vi "mod_Generate Histogram.vi"(0 "samples in":dbl[](array[numeric]) format="%.2f", 5 "max bin":dbl format="%.2f", 7 "min bin":dbl format="%.2f", 9 "bin size":dbl format="%.2f", 11 "error in (no error)":errorcluster, 13 "reset? (T)":bool=TRUE) -> (4 "histogram out":i32[](array[numeric]), 15 "error out":errorcluster)   [LabVIEW 2020, in "niAMT.lvlib"]
doc: "(c) Copyright 2006, National Instruments, Inc. This VI may not be duplicated, sold, or distributed without written consent from National Instruments."
uses:
  <vilib>/addons/Modulation/niAMT.lvlib
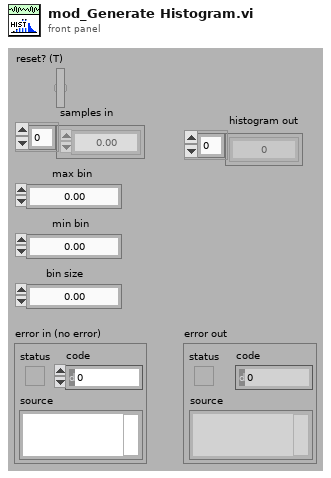
[diagram p1: front panel]
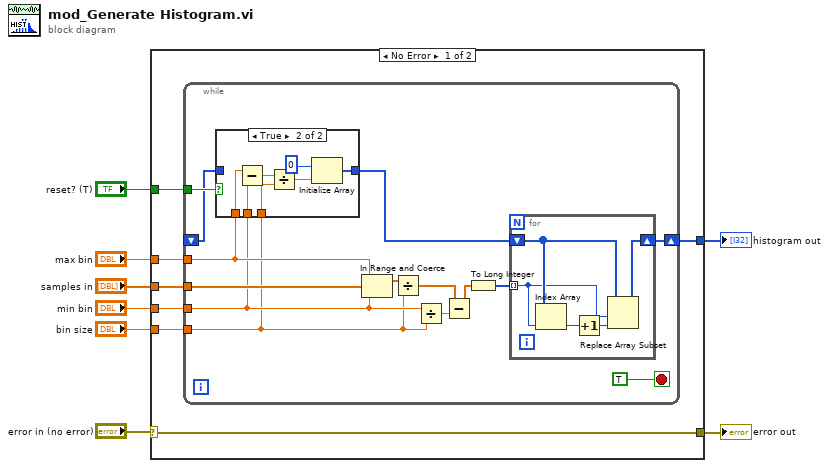
[diagram p0: block diagram]
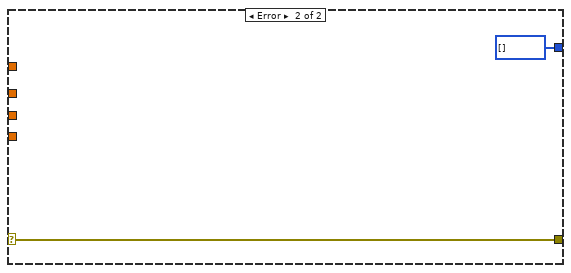
[diagram p3: hidden frame]
diagram:
  n1 = case shown="No Error" "error in (no error)" {
    selector: "error in (no error)" -> [w9 w44]
    tunnel: "samples in" -> [w15 _]
    tunnel: "min bin" -> [w14 _]
    tunnel: "max bin" -> [w13 _]
    tunnel: "bin size" -> [w12 _]
    tunnel: [w11 i32[] []] -> w4
    tunnel: "reset? (T)" -> [w10 _]
    tunnel: [w9 w44] -> w1
    frame No Error {
      n2 = while {
        tunnel: w15 -> [w29]
        tunnel: w14 -> [w20]
        tunnel: w13 -> [w21]
        tunnel: w12 -> [w19]
        shift-right: [w28] -> w11
        shift-left: _ -> [w17]
        tunnel: w10 -> [w22]
        stop <- TRUE stop-if-true
        n3 = case shown="True" w22 {
          tunnel: w21 -> [_ w34]
          tunnel: w20 -> [_ w33]
          tunnel: w19 -> [_ w32]
          tunnel: [w30 w31] -> w18
          tunnel: w17 -> [w30 _]
          frame False {
          }
          frame True {
            n4 = Subtract(x=w34, y=w33) -> (x-y=w36:dbl)
            n5 = Divide(x=w36, y=w32) -> (x/y=w35:dbl)
            n6 = Initialize Array(0 ("Numeric"), w35) -> (w31:i32[])
          }
        }
        n7 = In Range and Coerce(upper limit=w21, x=w29, lower limit=w20) -> (coerced(x)=w27:dbl[])  [unwired: 1 out]
        n8 = Divide(x=w27, y=w19) -> (x/y=w24:dbl[])
        n9 = Divide(x=w20, y=w19) -> (x/y=w25:dbl)
        n10 = Subtract(x=w24, y=w25) -> (x-y=w23:dbl[])
        n11 = To Long Integer(number=w23) -> (32bit integer=w26:i32[])
        n12 = for {
          tunnel: w26 -> [w38] mode=indexing
          shift-right: [w39] -> w28
          shift-left: w18 -> [w40]
          n13 = Index Array(array=w40, index=w38) -> (element=w42:i32)
          n14 = Increment(x=w42) -> (x+1=w41:i32)
          n15 = Replace Array Subset(array=w40, new element=w41, index=w38) -> (w39:i32[])
        }
      }
    }
    frame Error {
    }
  }
  "histogram out" <- w4
  "error out" <- w1
